vi "PathPlanner_GeomUtil_CalculateRadius.vi"(9 "C":T1 {"Y" format="%14.3f"; "X" format="%14.3f"}, 10 "B":T1 {"Y" format="%14.3f"; "X" format="%14.3f"}, 11 "A":T1 {"Y" format="%14.3f"; "X" format="%14.3f"}) -> (3 "Radius":dbl)   [LabVIEW 2019, in "PathPlanner24.lvlib"]
doc: "Calculate the curve radius given 3 points on the curve\n \nInputs: \n - a - translation2d - Point A\n - b - translation2d - Point B\n - c - translation2d - Point C\n\nOutputs:\n - Radius - double - Curve radius"
uses:
  PathPlanner24.lvlib
  <vilib>/Rock Robotics/WPI/ThirdParty/JAS_Junk/TrajLib/TypeDef/TRANSLATION2D.ctl
  <vilib>/Rock Robotics/WPI/ThirdParty/JAS_Junk/TrajLib/Util_CalcDist.vi
  <vilib>/Rock Robotics/WPI/ThirdParty/JAS_Junk/TrajLib/Translation2d_Create.vi
  <vilib>/Rock Robotics/WPI/ThirdParty/JAS_Junk/TrajLib/Trajectory_Library.lvlib
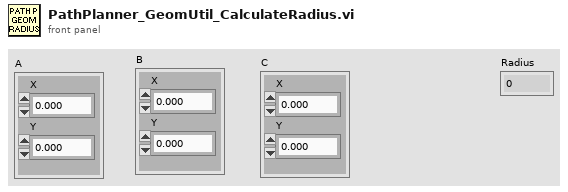
[diagram p1: front panel]
types:
  T1 = typedef "Trajectory_Library.lvlib/TRANSLATION2D.ctl" = cluster{"X":dbl, "Y":dbl}
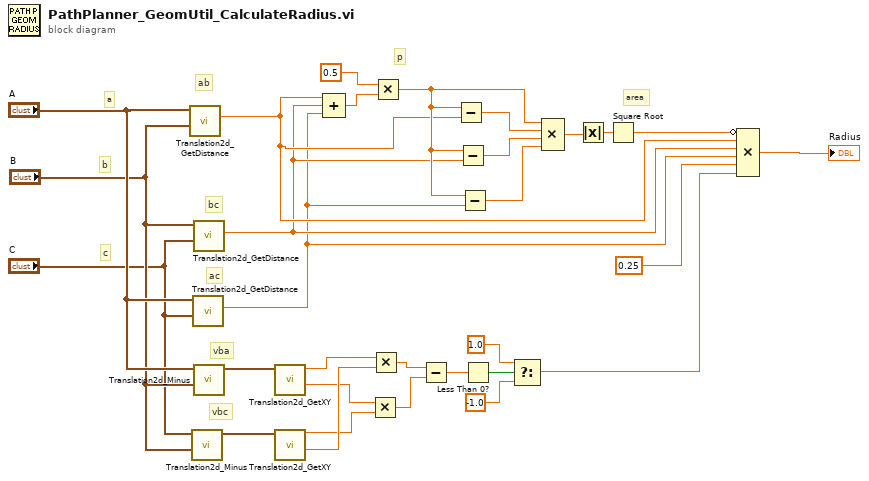
[diagram p0: block diagram]
diagram:
  # "vbc"
  # "vba"
  # "c"
  # "b"
  # "a"
  # "area"
  # "p"
  # "ac"
  # "bc"
  # "ab"
  n1 = call <vilib>:"Translation2d_GetDistance.vi"("other Translation"="B", "In Translation"="A") -> ("Distance"=w21:dbl)  [unwired: 9 in]
  n2 = call <vilib>:"Translation2d_Minus.vi"("other Translation"="B", "In Translation"="C") -> ("Out Translation"=w16:T1)  [unwired: 9 in]
  n3 = call <vilib>:"Translation2d_GetDistance.vi"("other Translation"="C", "In Translation"="A") -> ("Distance"=w19:dbl)  [unwired: 9 in]
  n4 = call <vilib>:"Translation2d_GetDistance.vi"("other Translation"="C", "In Translation"="B") -> ("Distance"=w20:dbl)  [unwired: 9 in]
  n5 = call <vilib>:"Translation2d_Minus.vi"("other Translation"="B", "In Translation"="A") -> ("Out Translation"=w17:T1)  [unwired: 9 in]
  n6 = call <vilib>:"Translation2d_GetXY.vi"("In Translation"=w17) -> ("Y"=w13:dbl, "X"=w15:dbl)  [unwired: 9 in]
  n7 = call <vilib>:"Translation2d_GetXY.vi"("In Translation"=w16) -> ("Y"=w14:dbl, "X"=w12:dbl)  [unwired: 9 in]
  n8 = Compound Arithmetic op=ADD(w21, w20, w19) -> (w30:dbl)
  n9 = Multiply(x=w13, y=w12) -> (x*y=w10:dbl)
  n10 = Multiply(x=w15, y=w14) -> (x*y=w11:dbl)
  n11 = Multiply(x=0.5, y=w30) -> (x*y=w28:dbl)
  n12 = Subtract(x=w11, y=w10) -> (x-y=w9:dbl)
  n13 = Subtract(x=w28, y=w21) -> (x-y=w27:dbl)
  n14 = Subtract(x=w28, y=w20) -> (x-y=w26:dbl)
  n15 = Subtract(x=w28, y=w19) -> (x-y=w25:dbl)
  n16 = Less Than 0?(x=w9) -> (x < 0?=w8:bool)
  n17 = Select(t=1.0, s=w8, f=-1.0) -> (s? t:f=w5:dbl)
  n18 = Compound Arithmetic op=MULTIPLY(w28, w27, w26, w25) -> (w24:dbl)
  n19 = Absolute Value(x=w24) -> (abs(x)=w23:dbl)
  n20 = Square Root(x=w23) -> (sqrt(x)=w22:dbl)
  n21 = Compound Arithmetic op=MULTIPLY(invert w22, w21, w20, w19, 0.25 ("value"), w5) -> (→"Radius":dbl)
